vi "9759 Constants and GUIDs.vi"() -> ()   [LabVIEW 2015, in "NI 9759 RevB Custom Device.lvlib"]
uses:
  NI 9759 RevB Custom Device.lvlib
  Types/Channel.ctl
panel:
  in  "Tab Control":enum32{"GUIDS", "Constants", "Chan Lists"}(tab)
  in  "GUID.Sect Write Del Prot":string="a1aa6f00-b9f7-40f6-887c-2c4f1e9d321e"
  in  "GUID.EnableDisable":string="77b71bdd-d372-4e98-a0cf-cacfe4ebb205"
  in  "GUID.Status":string="a24c8a18-6c61-49c1-a038-2eddd9d5ca1c"
  in  "GUID.Main Disabled":string="14ccdd51-a138-451a-a39a-671b6f30041d"
  in  "GUID.Sect Read Del Prot":string="7d62748c-5b5b-4fcc-a636-d9726e69d327"
  in  "GUID.Chan Del Prot":string="044eab8a-eaf9-4911-a08f-5455933789a0"
  in  "GUID.Main Enabled":string="043704e6-f96a-41ba-9f28-e0bf3582615c"
  in  "Constant.ConfirmDelete":string="Confirm delete configuration"
  in  "Constant.Diagnostics":string="Diagnostics"
  in  "Constant.Temperature":string="Temperature"
  in  "Constant.Invalid Selection":string="Invalid Selection"
  in  "Constant.Select":string="Select"
  in  "Constant.User OS":string="User OS"
  in  "Constant.Config":string="Config"
  in  "Constant.Input State":string="Input State"
  in  "Constant.Clear Faults":string="Clear Faults"
  in  "Constant.Debug":string="Debug"
  in  "Constant.System":string="System"
  in  "Constant.Description":string="Description"
  in  "Constant.Results":string="Results"
  in  "Constant.Setup":string="Setup"
  in  "Constant.Command":string="Command"
  in  "Constant.invalid bitfile":string="Invalid Bitfile"
  in  "Constant.ChangeBitfile":string="Changing bitfile will delete all relevant configuration information. Proceed?"
  in  "Constant.RemoveBitfile":string="Removing the bitfile path will delete all configuration information. Proceed?"
  in  "Constant.Status":string="Status"
  in  "Constant.Data":string="Data"
  in  "Constant.Control":string="Control"
  in  "Constant.not present":string="- not added -"
  in  "ChanList.Status Chans":T1[](array[typedef])=[{"Name"="Status code", "Units"="", "Default"=0.0, "Description"="Status code of the custom device. A negative value indicates failure. A positive value indicates warning."}, {"Name"="Loop duration", "Units"="ns", "Default"=0.0, "Description"="Duration of the custom device loop in nanoseconds. This can be monitored to measure performance relative to the desired loop rate."}, {"Name"="Late count", "Units"="", "Default"=0.0, "Description"="Number of times the custom device loop has gone late."}]
  in  "ChanList.9759 Data":T1[](array[typedef])=[{"Name"="TP1", "Units"="deg", "Default"=0.0, "Description"="Measured throttle position in degrees."}, {"Name"="TP2", "Units"="deg", "Default"=0.0, "Description"="Measured throttle position in degrees."}, {"Name"="Analog1", "Units"="V", "Default"=0.0, "Description"="Measured analog input in volts."}, {"Name"="Analog2", "Units"="V", "Default"=0.0, "Description"="Measured analog input in volts."}, {"Name"="ISense1", "Units"="A", "Default"=0.0, "Description"="Measured current in amps."}, {"Name"="ISense2", "Units"="A", "Default"=0.0, "Description"="Measured current in amps."}, {"Name"="Battery", "Units"="V", "Default"=0.0, "Description"="Measured battery voltage supplied to the module."}, {"Name"="Temperature", "Units"="C", "Default"=0.0, "Description"="Measured temperature inside the module."}, {"Name"="ModulePresent", "Units"="bool", "Default"=0.0, "Description"="Indicates that the module has been found in the specified slot and is powered."}, {"Name"="Fault1", "Units"="bool", "Default"=0.0, "Description"="Indicates a fault on the specified channel."}, {"Name"="Fault2", "Units"="bool", "Default"=0.0, "Description"="Indicates a fault on the specified channel."}]
  in  "ChanList.9759 Controls":T1[](array[typedef])=[{"Name"="ModuleEnable", "Units"="bool", "Default"=0.0, "Description"="Enables module functionality."}, {"Name"="ControlEnable1", "Units"="bool", "Default"=0.0, "Description"="Enables channel output."}, {"Name"="ControlEnable2", "Units"="bool", "Default"=0.0, "Description"="Enables channel output."}, {"Name"="Setpoint1", "Units"="deg", "Default"=0.0, "Description"="Desired position setpoint in degrees."}, {"Name"="Setpoint2", "Units"="deg", "Default"=0.0, "Description"="Desired position setpoint in degrees."}]
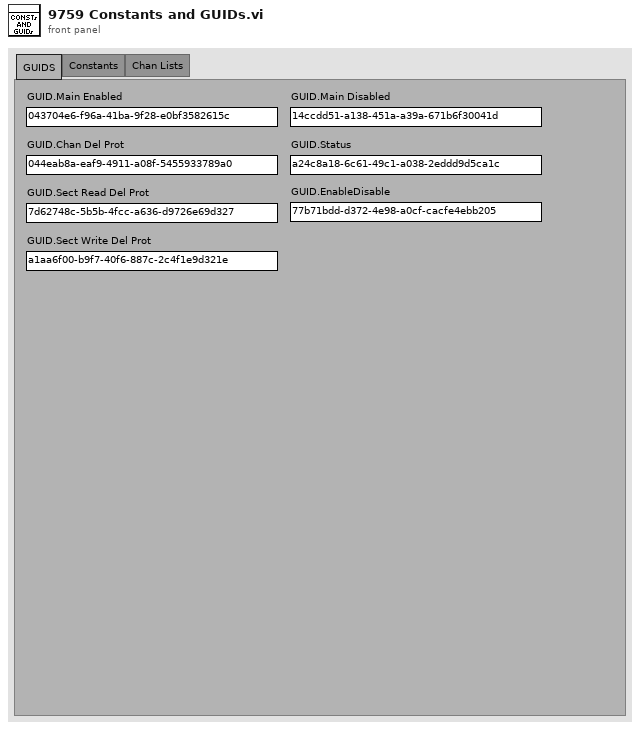
[diagram p1: front panel]
types:
  T1 = typedef "NI 9759 RevB Custom Device.lvlib/Channel.ctl" = cluster{"Name":string, "Units":string, "Default":dbl, "Description":string}
diagram:
